vi "remove_instance.vi"(8 "error in (no error)":errorcluster, 9 "Object Instance":refnum<data-value>, 10 "Base Class (LabVIEW Object)":refnum<class>, 11 "Default Lookup in":refnum<class "Default Lookup.lvclass">) -> (0 "error out":errorcluster, 1 "removed?":bool, 3 "Default Lookup out":refnum<class "Default Lookup.lvclass">)   [LabVIEW 2014, in "LVCOOOP.lvlib" / "Lookup API.lvlib" / "Default Lookup.lvclass"]
uses:
  Default Lookup.lvclass
  Default Lookup.lvclass/Default Lookup.ctl
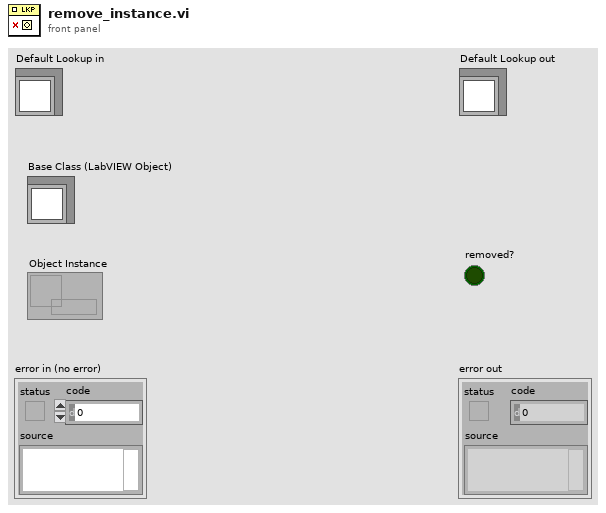
[diagram p1: front panel]
types:
  T1 = typedef "LVCOOOP.lvlib/Lookup API.lvlib/Default Lookup.lvclass/lookup_data.ctl" = cluster{"instances":refnum<data-value>[], "listeners":refnum<user-event>[]}
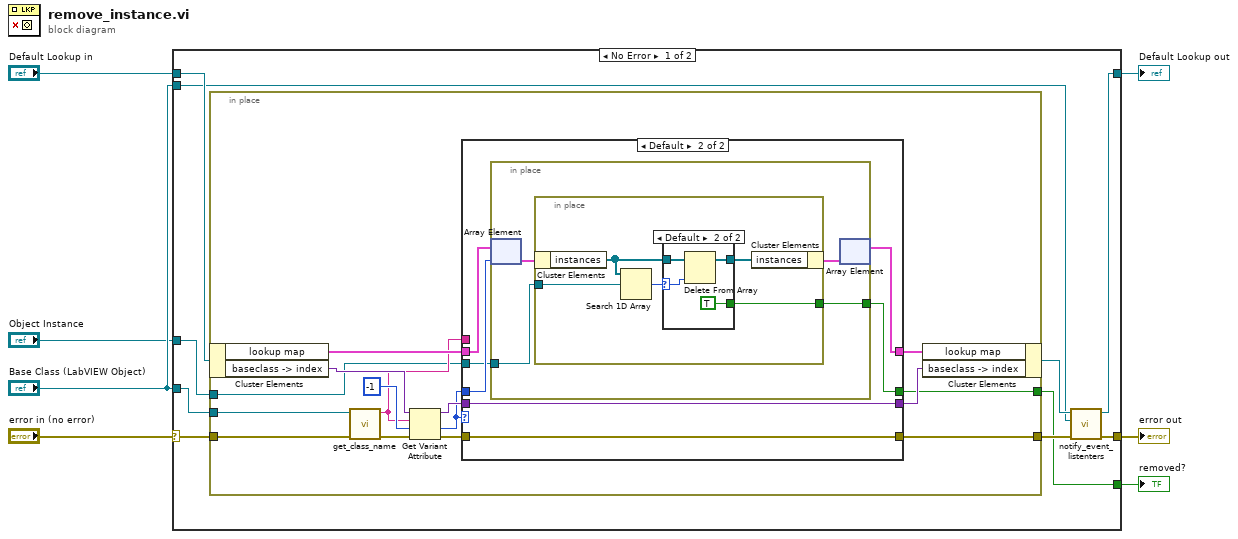
[diagram p0: block diagram]
diagram:
  n1 = case shown="No Error" "error in (no error)" {
    selector: "error in (no error)" -> [w15 w57]
    tunnel: "Default Lookup in" -> [w17 w58]
    tunnel: "Base Class (LabVIEW Object)" -> [w16 _]
    tunnel: [w11 w58] -> w5
    tunnel: [w12 w57] -> w6
    tunnel: "Base Class (LabVIEW Object)" -> [w10 _]
    tunnel: "Object Instance" -> [w9 _]
    tunnel: [w8 _] -> w1
    frame No Error {
      n2 = in-place {
        in-place-border: w16 -> [w31]
        in-place-border: w15 -> [w30]
        in-place-border: [w20] -> w13
        in-place-border: w9 -> [w19]
        in-place-border: [w18] -> w8
        n3 = in-place-cluster #1(w17) -> ("lookup map"=w27:T1[], "baseclass -> index"=w32:variant)
        n4 = call "get_class_name.vi"("error in (no error)"=w30, "LabVIEW Object in"=w31) -> ("error out"=w29:errorcluster, "class name"=w24:string)  [unwired: 8 in]
        n5 = Get Variant Attribute(Variant=w32, name=w24, default value (empty Variant)=-1, error in=w29) -> (duplicate Variant=w25:variant, value=w21:i32, error out=w23:errorcluster)  [unwired: 1 out]
        n6 = case shown="Default" w21 {
          tunnel: w27 -> [w35 w42]
          tunnel: [w35 w41] -> w26
          tunnel: w25 -> [w34 w39]
          tunnel: w24 -> [_ _]
          tunnel: w23 -> [w33 w38]
          tunnel: [w34 w39] -> w22
          tunnel: w21 -> [_ w40]
          tunnel: [w33 w38] -> w20
          tunnel: w19 -> [_ w37]
          tunnel: [_ w36] -> w18
          frame -1 {
          }
          frame Default {
            n7 = in-place {
              in-place-border: w37 -> [w44]
              in-place-border: [w43] -> w36
              n8 = in-place-array #2(w42, w40) -> (w46:T1)
              n9 = in-place {
                in-place-border: w44 -> [w51]
                in-place-border: [w47] -> w43
                n10 = in-place-cluster #3(w46) -> ("instances"=w50:refnum<data-value>[])
                n11 = Search 1D Array(1D array=w50, element=w51) -> (index of element=w48:i32)  [unwired: 1 in]
                n12 = case shown="Default" w48 {
                  selector: w48 -> [_ w54]
                  tunnel: w50 -> [w52 w56]
                  tunnel: [w52 w55] -> w49
                  tunnel: [_ TRUE] -> w47
                  frame -1 {
                  }
                  frame Default {
                    n13 = Delete From Array(array=w56, index=w54) -> (array with subset deleted=w55:refnum<data-value>[])  [unwired: 1 in, 1 out]
                  }
                }
                n14 = in-place-cluster #3("instances"=w49) -> (w45:T1)
              }
              n15 = in-place-array #2(w45) -> (w41:T1[])  [unwired: 1 out]
            }
          }
        }
        n16 = in-place-cluster #1("lookup map"=w26, "baseclass -> index"=w22) -> (w14:refnum<class "Default Lookup.lvclass">)
      }
      n17 = call-dynamic "notify_event_listenters.vi"("error in (no error)"=w13, "Base Class (LabVIEW Object)"=w10, "Default Lookup in"=w14) -> ("error out"=w12:errorcluster, "Default Lookup out"=w11:refnum<class "Default Lookup.lvclass">)  [unwired: 7 in]
    }
    frame Error {
    }
  }
  "error out" <- w6
  "Default Lookup out" <- w5
  "removed?" <- w1
